vi "FPGA_main.vi"() -> ()   [LabVIEW 2020]
uses:
  #typedef_accelerations.ctl
  #typedef_FPGA_States.ctl
  <vilib>/Platform/TimedLoop/XDataNode/timing_clust.ctl
  <vilib>/Platform/TimedLoop/XDataNode/nitl_modes.ctl
  <vilib>/Platform/TimedLoop/XDataNode/wakeup.ctl
  <vilib>/rvi/Emulation/niFpgaGetClockAttributes.vi
  <vilib>/rvi/Emulation/niFpgaSctlEmulationGetInTimedLoop.vi
  <vilib>/rvi/Emulation/niFpgaEmulationReportErrorSimple.vi
  <vilib>/rvi/Emulation/niFpgaEmulationIsFPGAContextNoSignature.vi
  <vilib>/rvi/DataTransferAndStorage/Container/Common/niFpgaContainerGetUniqueNameForEmu.vi
  <vilib>/rvi/Memory/Memory_Emulation/niFpgaMemoryEmulationCacheClearOnFirstRun.vi
  <vilib>/rvi/Memory/Memory_Emulation/nirvimemoryEmulationManagerCache_MakeExclusive.vi
  <vilib>/rvi/Memory/Memory_Emulation/niFpgaMemoryEmulationValidateCache.vi
  <vilib>/rvi/Memory/Memory_Emulation/nirvimemoryEmulationManagerCache_InsertValue.vi
  <vilib>/Utility/error.llb/Clear Errors.vi
  <vilib>/rvi/Memory/Memory_Emulation/nirvimemoryEmulationManagerCache_ReleaseExclusive.vi
  <vilib>/rvi/Memory/Memory_Emulation/nirvimemoryEmulationManagerCache_GetValue.vi
  <vilib>/rvi/Memory/Memory_Emulation/nirvimemoryEmulationManagerCache_SetValue.vi
  <vilib>/rvi/Emulation/niFpgaProcessEmulError.vi
  <vilib>/rvi/eio/common/nirviEmuTemplateMethod_errors.vi
  <vilib>/rvi/Emulation/niFpgaCriticalErrorInLSC.vi
  <vilib>/rvi/errors/niFpgaSetErrorForExecOnDevCompSimple.vi
  <vilib>/rvi/eio/common/nirviEmuReportErrorAndStop.vi
  <vilib>/rvi/FIFO/Fifo_Resource/nirvififoEmulationSetSize.vi
  <vilib>/rvi/FIFO/Fifo_Resource/nirviFifoEmulationQueueMgr.vi
  <instcachedir>/0/nirviFifoEmulationQueueMgr_E5CAEC123FF24DC58D834DCA3CDAA9B5.lvgen/nirviFifoEmulationQueueMgr_E5CAEC123FF24DC58D834DCA3CDAA9B5_001.vi
  <vilib>/rvi/FIFO/Fifo_Resource/nirvififoEmulationDetermineInputValidOut.vi
  <vilib>/rvi/FIFO/Fifo_Resource/nirvififoEmulationCreateLock.vi
  <vilib>/rvi/FIFO/Fifo_Resource/nirvififoEmulationObtainLock.vi
  <vilib>/rvi/FIFO/Fifo_Resource/nirvififoEmulationReleaseLock.vi
  <vilib>/rvi/occurrence/nirviWaitOnOccurrenceBase.vi
  <vilib>/rvi/errors/nirviReportUnexpectedCaseInternalError.vi
  <vilib>/rvi/errors/nirviReportUnexpectedCaseInternalError (U32).vi
  <vilib>/rvi/Memory/Memory_Emulation/nirvimemoryFastEmulation.vi
  <vilib>/rvi/Memory/Memory_Emulation/nirvimemoryEmulation.vi
  <vilib>/rvi/interface/RandomDataEmulation/niFpgaRandomDataHandleErrors.vi
  <vilib>/rvi/DataTransferAndStorage/Container/XNode/niFpgaContainer.xnode
  <vilib>/rvi/DataTransferAndStorage/Register/Emulation/niFpgaRegisterEmulation.vi
  <vilib>/eio/EIONode/EIONode.xnode
  <vilib>/platform/TimedLoop/XDataNode/XDataNode.xnode
  <vilib>/rvi/FIFO/Fifo_Resource/nirvififoEmulationWrite.vi
  <vilib>/rvi/DataTransferAndStorage/Handshake/Emulation/niFpgaHandshakeEmulation.vi
  <vilib>/rvi/FIFO/Fifo_Resource/nirvififoEmulationRead.vi
  <vilib>/rvi/interface/RandomDataEmulation/nirviRandomDataFpgaReadWriteTemplate.vi
  <vilib>/Platform/TimedLoop/XDataNode/XDNodeRunTimeDep.lvlib
panel:
  in  "PostTriggerDataLength":u16
  in  "PreTriggerDataLength":u16
  in  "stop":bool
  in  "Monitoring?":bool
  in  "TriggerZ":i16
  in  "TriggerY":i16
  in  "SamplesOverThreshold (<255)":u8
  in  "TriggerX":i16
  in  "Acceleration":T1
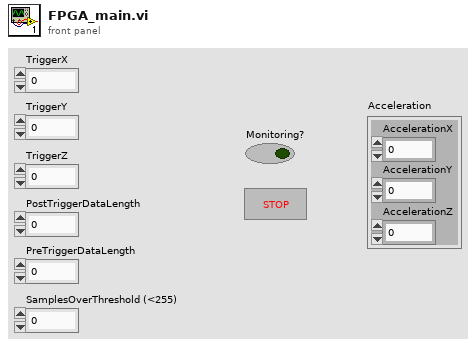
[diagram p1: front panel]
types:
  T1 = typedef "#typedef_accelerations.ctl" = cluster{"AccelerationX":i16, "AccelerationY":i16, "AccelerationZ":i16}
  T2 = typedef "#typedef_FPGA_States.ctl" = enum16{"Idle", "Monitoring", "SendPreTriggerData", "SendPostTriggerData"}
  T3 = typedef "XDNodeRunTimeDep.lvlib/timing_clust.ctl" = cluster{"Expected End [f-1]":u64, "Actual End [f-1]":u64, "Finished Late? [f-1]":bool, "Expected End [i-1]":u64, "Actual End [i-1]":u64, "Finished Late? [i-1]":bool, "Expected Start [i]":u64, "Actual Start [i]":u64, "Expected Start [f]":u64, "Actual Start [f]":u64, "Source Name":string, "Structure Name":string, "Period":i64, "Deadline":i64, "Offset":i64, "Start":i64, "Priority":i32, "Timeout":i32, "Mode":T4, "Wakeup Reason":T5, "Error":errorcluster, "Source Type":string, "Secondary Source Type":string, "Global End Time":u64, "Global Start Time":u64, "Frame Duration":u64, "Iteration Duration":u64, "Assigned CPU":i32, "I/O Scan Engine Mode":u32}
  T4 = typedef "XDNodeRunTimeDep.lvlib/nitl_modes.ctl" = enum32{"No Change", "Process missed periods, maintain original phase", "Discard missed periods, maintain original phase", "Process missed periods, ignore original phase", "Discard missed periods, ignore original phase"}
  T5 = typedef "XDNodeRunTimeDep.lvlib/wakeup.ctl" = enum32{"Normal", "Aborted", "Asynchronous wakeup", "Timing source error", "Timed loop error", "Timeout"}
  T6 = cluster{"AccelerationX":i16, "AccelerationY":i16, "AccelerationZ":i16}
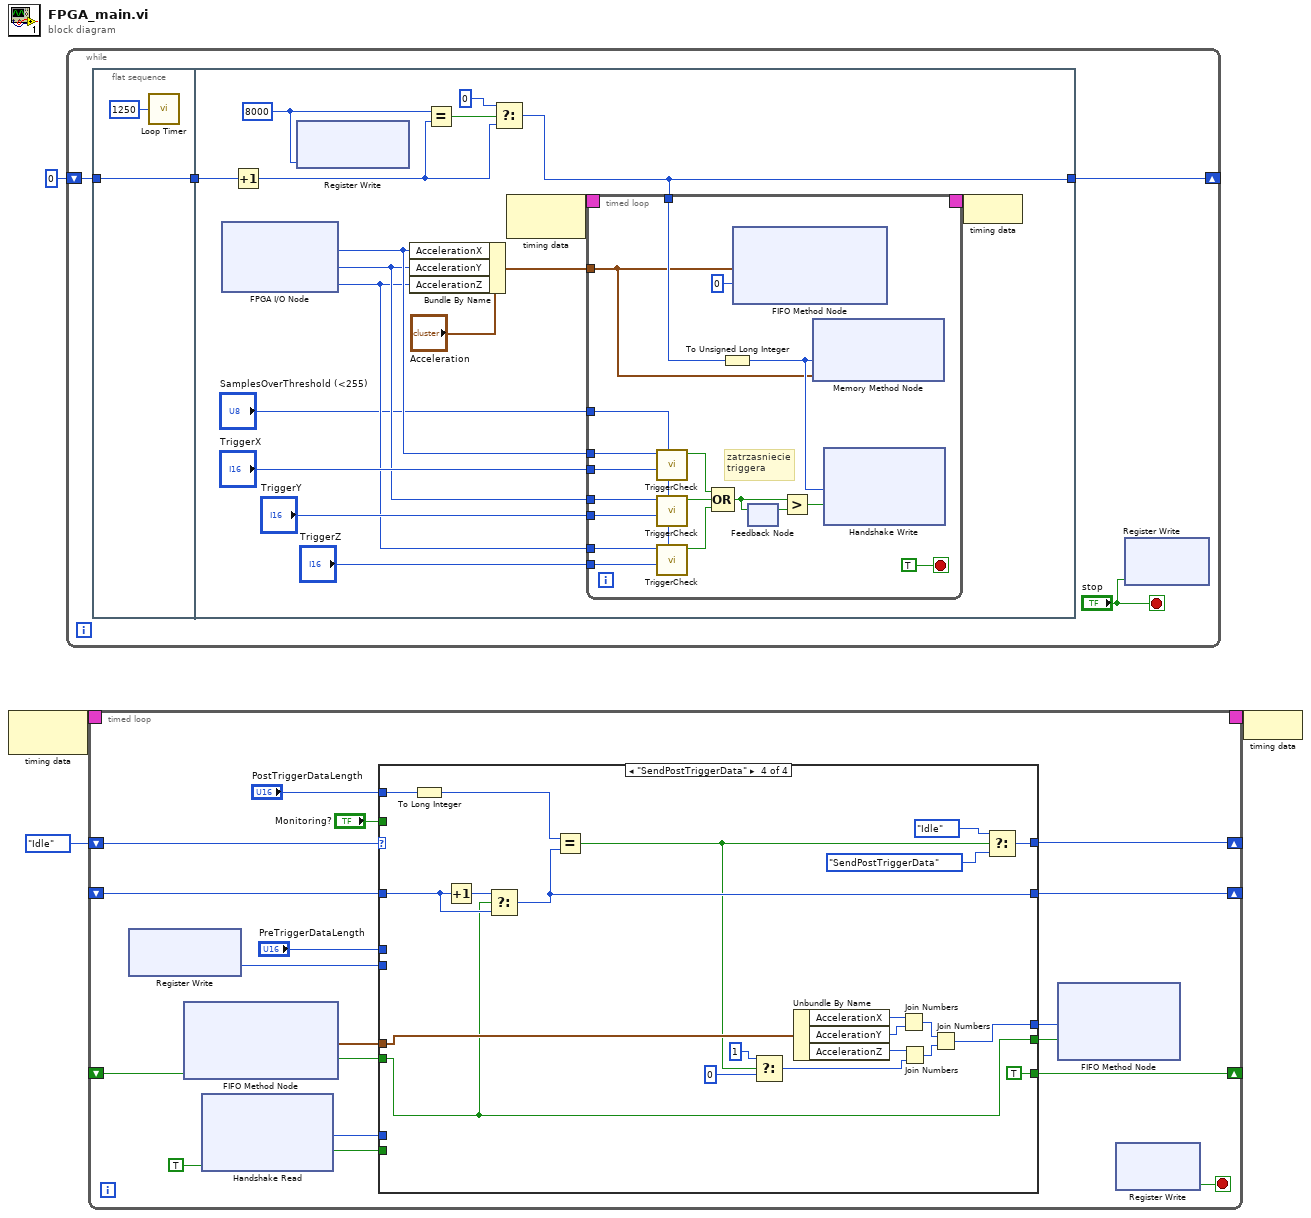
[diagram p0: block diagram]
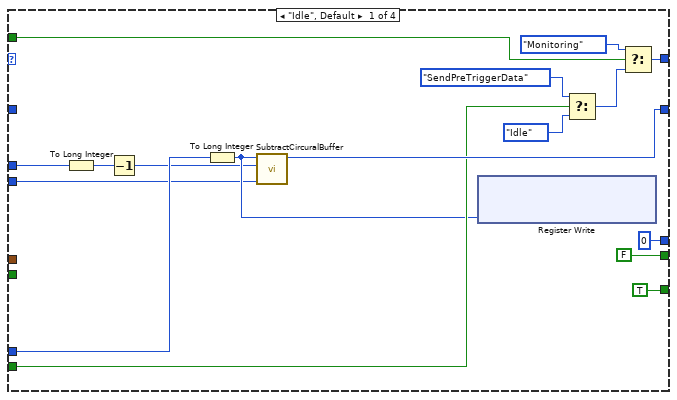
[diagram p2: hidden frame]
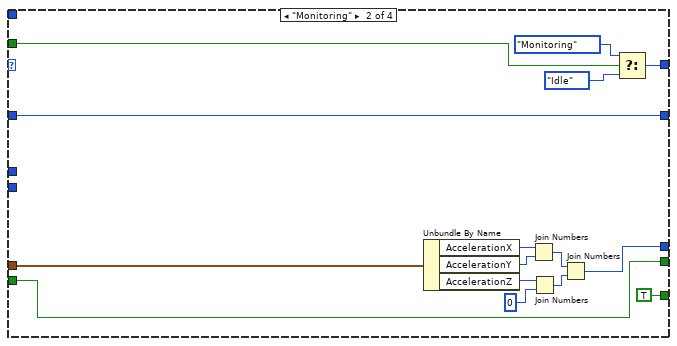
[diagram p3: hidden frame]
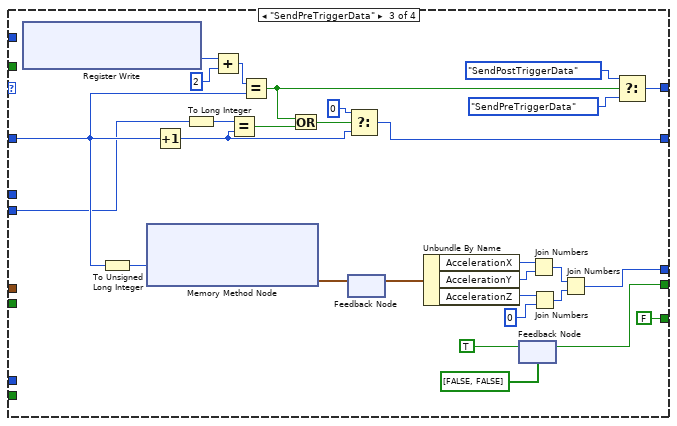
[diagram p4: hidden frame]
diagram:
  n1 = node-c288() -> (w3:T3)  [unwired: 1 in]
  n2 = while {
    shift-right: [w6] -> _
    shift-left: u16 0 -> [w8]
    stop <- "stop" stop-if-true
    n3 = flat-sequence {
      tunnel: w8 -> [w9]
      tunnel: [w9] -> w7
      tunnel: w7 -> [w26]
      tunnel: [w22] -> w6
      frame #0 {
        n4 = call "Loop Timer"("Count(uSec)"=u16 1250) -> ()  [unwired: 1 out]
      }
      frame #1 {
        w11 = u16 8000 ("x")
        n5 = xnode "FPGA I/O Node"() -> ("AccelerationX"=w21:i16, "AccelerationY"=w17:i16, "AccelerationZ"=w16:i16)  [unwired: 3 in, 3 out]
        n6 = Increment(x=w26) -> (x+1=w23:u16)
        n7 = xnode "Register Write"("Data"=w11) -> ()  [unwired: 1 in, 1 out]
        n8 = Bundle By Name(cluster="Acceleration", "AccelerationX"=w21, "AccelerationY"=w17, "AccelerationZ"=w16) -> (w15:T1)
        n9 = Equal?(x=w11, y=w23) -> (x = y?=w25:bool)
        n10 = Select(t=u16 0, s=w25, f=w23) -> (s? t:f=w22:u16)
        n11 = node-c288() -> (w14:T3)  [unwired: 1 in]
        n12 = timed-loop {
          timing: w14 -> [_]
          timing-out: [_] -> w13
          tunnel: w22 -> [w45]
          tunnel: w21 -> [w44]
          tunnel: "TriggerX" -> [w43]
          tunnel: "SamplesOverThreshold (<255)" -> [w42]
          tunnel: "TriggerY" -> [w41]
          tunnel: "TriggerZ" -> [w40]
          tunnel: w17 -> [w39]
          tunnel: w16 -> [w38]
          tunnel: w15 -> [w29]
          stop <- TRUE stop-if-true
          # "zatrzasniecie\ntriggera"
          n13 = call "TriggerCheck.vi"("SamplesOverThreshold (<255)"=w42, "TriggerLevel"=w43, "Acceleration"=w44) -> ("Trigger?"=w36:bool)  [unwired: 8 in]
          n14 = call "TriggerCheck.vi"("SamplesOverThreshold (<255)"=w42, "TriggerLevel"=w41, "Acceleration"=w39) -> ("Trigger?"=w37:bool)  [unwired: 8 in]
          n15 = call "TriggerCheck.vi"("SamplesOverThreshold (<255)"=w42, "TriggerLevel"=w40, "Acceleration"=w38) -> ("Trigger?"=w35:bool)  [unwired: 8 in]
          n16 = Compound Arithmetic op=OR(w36, w37, w35) -> (w32:bool)
          n17 = To Unsigned Long Integer(number=w45) -> (unsigned 32bit integer=w30:u32)
          n18 = xnode ("FIFO Method Node")("Element"=w29, "Timeout"=0) -> ()  [unwired: 1 in, 2 out]
          n19 = feedback-in #1(w32) -> ()
          n20 = feedback #1() -> (w33:bool)  [unwired: 1 in]
          n21 = Greater?(x=w32, y=w33) -> (0:w31:bool)
          n22 = xnode ("Memory Method Node")("Address"=w30, "Data"=w29) -> ()  [unwired: 1 in, 1 out]
          n23 = xnode "Handshake Write"("Data"=w30, "Input Valid"=w31) -> ()  [unwired: 1 in, 2 out]
        }
        n24 = node-c288(w13) -> ()
      }
    }
    n25 = xnode "Register Write"("Data"="stop") -> ()  [unwired: 1 in, 1 out]
  }
  n26 = timed-loop {
    timing: w3 -> [_]
    timing-out: [_] -> w2
    shift-right: [w66] -> _
    shift-left: #typedef_FPGA_States."Idle" -> [w67]
    shift-right: [w51] -> _
    shift-left: _ -> [w61]
    shift-right: [w53] -> _
    shift-left: _ -> [w54]
    stop <- w62 stop-if-true
    n27 = xnode "Register Write"() -> ("Data"=w50:u16)  [unwired: 1 in, 1 out]
    n28 = xnode ("FIFO Method Node")("Ready for Output"=w54) -> ("Element"=w58:T6, "Output Valid"=w52:bool)  [unwired: 1 in, 1 out]
    n29 = xnode "Handshake Read"("Ready for Output"=TRUE) -> ("Data"=w55:u32, "Output Valid"=w56:bool)  [unwired: 1 in, 1 out]
    n30 = case shown="\"SendPostTriggerData\"" w67 {
      tunnel: [w84 w96 w126 w147] -> w66
      tunnel: "Monitoring?" -> [w79 w99 _ _]
      tunnel: [u64 0 w89 w111 w141] -> w64
      tunnel: [FALSE w85 w106 w130] -> w63
      tunnel: w61 -> [_ w88 w112 w136]
      tunnel: [w75 w88 w113 w135] -> w51
      tunnel: "PreTriggerDataLength" -> [w76 _ _ _]
      tunnel: "PostTriggerDataLength" -> [_ _ _ w140]
      tunnel: w58 -> [_ w87 _ w138]
      tunnel: w56 -> [w74 _ _ _]
      tunnel: w55 -> [w73 _ _ _]
      tunnel: [TRUE TRUE FALSE TRUE] -> w53
      tunnel: w52 -> [_ w85 _ w130]
      tunnel: w50 -> [w68 _ w101 _]
      frame "Idle", Default {
        n31 = To Long Integer(number=w76) -> (32bit integer=w72:i32)
        n32 = Decrement(x=w72) -> (x-1=w69:i32)
        n33 = To Long Integer(number=w73) -> (32bit integer=w71:i32)
        n34 = call "SubtractCircuralBuffer.vi"("BufferLength"=w68, "y"=w69, "x"=w71) -> ("z"=w75:i32)  [unwired: 8 in]
        n35 = xnode "Register Write"("Data"=w71) -> ()  [unwired: 1 in, 1 out]
        n36 = Select(t=#typedef_FPGA_States."SendPreTriggerData", s=w74, f=#typedef_FPGA_States."Idle") -> (s? t:f=w82:T2)
        n37 = Select(t=#typedef_FPGA_States."Monitoring", s=w79, f=w82) -> (s? t:f=w84:T2)
      }
      frame "Monitoring" {
        n38 = Unbundle By Name(w87) -> ("AccelerationX"=w95:i16, "AccelerationY"=w94:i16, "AccelerationZ"=w93:i16)
        n39 = Join Numbers(hi=w95, lo=w94) -> ((hi.lo)=w91:u32)
        n40 = Join Numbers(hi=w93, lo=i16 0) -> ((hi.lo)=w90:u32)
        n41 = Join Numbers(hi=w91, lo=w90) -> ((hi.lo)=w89:u64)
        n42 = Select(t=#typedef_FPGA_States."Monitoring", s=w99, f=#typedef_FPGA_States."Idle") -> (s? t:f=w96:T2)
      }
      frame "SendPreTriggerData" {
        n43 = xnode "Register Write"() -> ("Data"=w116:i32)  [unwired: 1 in, 1 out]
        n44 = To Unsigned Long Integer(number=w112) -> (unsigned 32bit integer=w117:u32)
        n45 = xnode ("Memory Method Node")("Address"=w117) -> ("Data"=w119:T6)  [unwired: 1 in, 1 out]
        n46 = Increment(x=w112) -> (x+1=w115:i32)
        n47 = To Long Integer(number=w101) -> (32bit integer=w100:i32)
        n48 = Add(x=w116, y=2) -> (x+y=w104:i32)
        n49 = Equal?(x=w100, y=w115) -> (x = y?=w109:bool)
        n50 = Equal?(x=w104, y=w112) -> (x = y?=w110:bool)
        n51 = Or(x=w110, y=w109) -> (x .or. y?=w108:bool)
        n52 = feedback-in #2(w119) -> ()
        n53 = feedback #2() -> (w107:T6)  [unwired: 1 in]
        n54 = Select(t=0, s=w108, f=w115) -> (s? t:f=w113:i32)
        n55 = Unbundle By Name(w107) -> ("AccelerationX"=w125:i16, "AccelerationY"=w124:i16, "AccelerationZ"=w123:i16)
        n56 = feedback-in #3(TRUE ("Output Valid")) -> ()
        n57 = feedback #3(bool[] [FALSE, FALSE]) -> (w106:bool)
        n58 = Join Numbers(hi=w125, lo=w124) -> ((hi.lo)=w121:u32)
        n59 = Join Numbers(hi=w123, lo=i16 0) -> ((hi.lo)=w120:u32)
        n60 = Join Numbers(hi=w121, lo=w120) -> ((hi.lo)=w111:u64)
        n61 = Select(t=#typedef_FPGA_States."SendPostTriggerData", s=w110, f=#typedef_FPGA_States."SendPreTriggerData") -> (s? t:f=w126:T2)
      }
      frame "SendPostTriggerData" {
        n62 = To Long Integer(number=w140) -> (32bit integer=w139:i32)
        n63 = Increment(x=w136) -> (x+1=w137:i32)
        n64 = Select(t=w137, s=w130, f=w136) -> (s? t:f=w135:i32)
        n65 = Equal?(x=w139, y=w135) -> (x = y?=w134:bool)
        n66 = Select(t=i16 1, s=w134, f=i16 0 ("lo")) -> (s? t:f=w131:i16)
        n67 = Unbundle By Name(w138) -> ("AccelerationX"=w146:i16, "AccelerationY"=w145:i16, "AccelerationZ"=w144:i16)
        n68 = Join Numbers(hi=w146, lo=w145) -> ((hi.lo)=w143:u32)
        n69 = Join Numbers(hi=w144, lo=w131) -> ((hi.lo)=w142:u32)
        n70 = Join Numbers(hi=w143, lo=w142) -> ((hi.lo)=w141:u64)
        n71 = Select(t=#typedef_FPGA_States."Idle", s=w134, f=#typedef_FPGA_States."SendPostTriggerData") -> (s? t:f=w147:T2)
      }
    }
    n72 = xnode ("FIFO Method Node")("Element"=w64, "Input Valid"=w63) -> ()  [unwired: 1 in, 2 out]
    n73 = xnode "Register Write"() -> ("Data"=w62:bool)  [unwired: 1 in, 1 out]
  }
  n74 = node-c288(w2) -> ()
